vi "总磷总氮测量数据储存.vi"   [LabVIEW 2016, in "斯坦道氨氮V2.lvlib"]
uses:
  <vilib>/ptbypt/NI_PtbyPt.lvlib
types:
  T1 = cluster{"跨度值":dbl, "零点标准液浓度":dbl, "跨度标准液浓度":dbl, "标准液标准浓度":dbl}
  T2 = cluster{"系统时间":timestamp, "工作状态":u16, "测量模式":enum16{"待机", "连续模式", "周期模式", "定点模式", "受控模式", "手动模式"}, "告警代码":u16, "故障代码":u16, "日志代码":u16, "软件版本":u16, "F0":sgl, "F1":sgl, "F2":sgl, "F3":sgl, "T":sgl, "H":sgl, "id":u16, "flowid":u16, "量程":u16, "总磷控温温度1":sgl, "营养盐控温温度2":sgl, "ADC":sgl}
  T3 = cluster{"运行模式":enum16{"维护模式", "常规模式", "应急模式", "质控模式"}, "质控频次":enum16{"关闭", "每天", "星期一", "星期二", "星期三", "星期四", "星期五", "星期六", "星期日"}, "空白核查时间":u16, "跨度核查时间":u16, "测量间隔":dbl}
  T4 = cluster{"总磷跨度值":dbl, "总磷零点标准液浓度":dbl, "总磷跨度标准液浓度":dbl, "总磷标准液标准浓度":dbl, "总氮跨度值":dbl, "总氮零点标准液浓度":dbl, "总氮跨度标准液浓度":dbl, "总氮标准液标准浓度":dbl, "氨氮跨度值":dbl, "氨氮零点标准液浓度":dbl, "氨氮跨度标准液浓度":dbl, "氨氮标准液标准浓度":dbl}
  T5 = cluster{"因子编码":u32, "单位":u16, "标样参考值":sgl, "水样数据时间":timestamp, "水样实测值":sgl, "水样数据标识":string, "标样数据时间":timestamp, "标样实测值":sgl, "标样数据标识":string, "空白数据时间":timestamp, "空白实测值":sgl, "空白数据标识":string, "零点核查数据时间":timestamp, "零点核查实测值":sgl, "零点核查数据标识":string, "跨度核查数据时间":timestamp, "跨度核查实测值":sgl, "跨度核查数据标识":string, "加标回收数据时间":timestamp, "加标回收实测值":sgl, "加标回收数据标识":string, "平行样数据时间":timestamp, "平行样实测值":sgl, "平行样数据标识":string, "F0":sgl, "F1":sgl, "F2":sgl, "F3":sgl, "F4":sgl, "F5":sgl, "F6":sgl, "F7":sgl, "温度":sgl, "湿度":sgl, "X值":sgl, "fidrange":u16}[]
  T6 = cluster{"因子编码":u32, "单位":u16, "标样参考值":sgl, "水样数据时间":timestamp, "水样实测值":sgl, "水样数据标识":string, "标样数据时间":timestamp, "标样实测值":sgl, "标样数据标识":string, "空白数据时间":timestamp, "空白实测值":sgl, "空白数据标识":string, "零点核查数据时间":timestamp, "零点核查实测值":sgl, "零点核查数据标识":string, "跨度核查数据时间":timestamp, "跨度核查实测值":sgl, "跨度核查数据标识":string, "加标回收数据时间":timestamp, "加标回收实测值":sgl, "加标回收数据标识":string, "平行样数据时间":timestamp, "平行样实测值":sgl, "平行样数据标识":string, "F0":sgl, "F1":sgl, "F2":sgl, "F3":sgl, "F4":sgl, "F5":sgl, "F6":sgl, "F7":sgl, "温度":sgl, "湿度":sgl, "X值":sgl, "fidrange":u16}
  T7 = cluster{"时间标识":timestamp, "测量模式":enum16{"维护数据", "水样测试", "标样核查", "零点核查", "跨度核查", "空白测试", "平行样测试", "加标回收", "空白校准", "标样校准", "初始化（清洗）", "快捷测试"}, "数据标记表":string, "监测值":sgl, "单位":u16, "数据标识":string, "因子编码":u32, "标样参考值":sgl, "F0":sgl, "F1":sgl, "F2":sgl, "F3":sgl, "F4":sgl, "F5":sgl, "F6":sgl, "F7":sgl, "X":sgl, "温度":sgl, "湿度":sgl, "量程标识":string, "SN":string, "跨度值":sgl, "X1":sgl}
  T8 = typedef "斯坦道氨氮V2.lvlib/关键参数.ctl" = cluster{"测量量程":sgl, "测量检出限":sgl, "测量精度":sgl, "测量间隔":sgl, "消解温度":sgl, "消解时长":sgl, "三项式系数":sgl, "二次多项式系数":sgl, "曲线斜率":sgl, "曲线截距":sgl, "线性相关系数":sgl, "空白校准时间":timestamp, "标样校准时间":timestamp, "测量信号值":sgl, "稀释倍数":sgl, "空白标定系数":sgl, "量程系数":sgl}
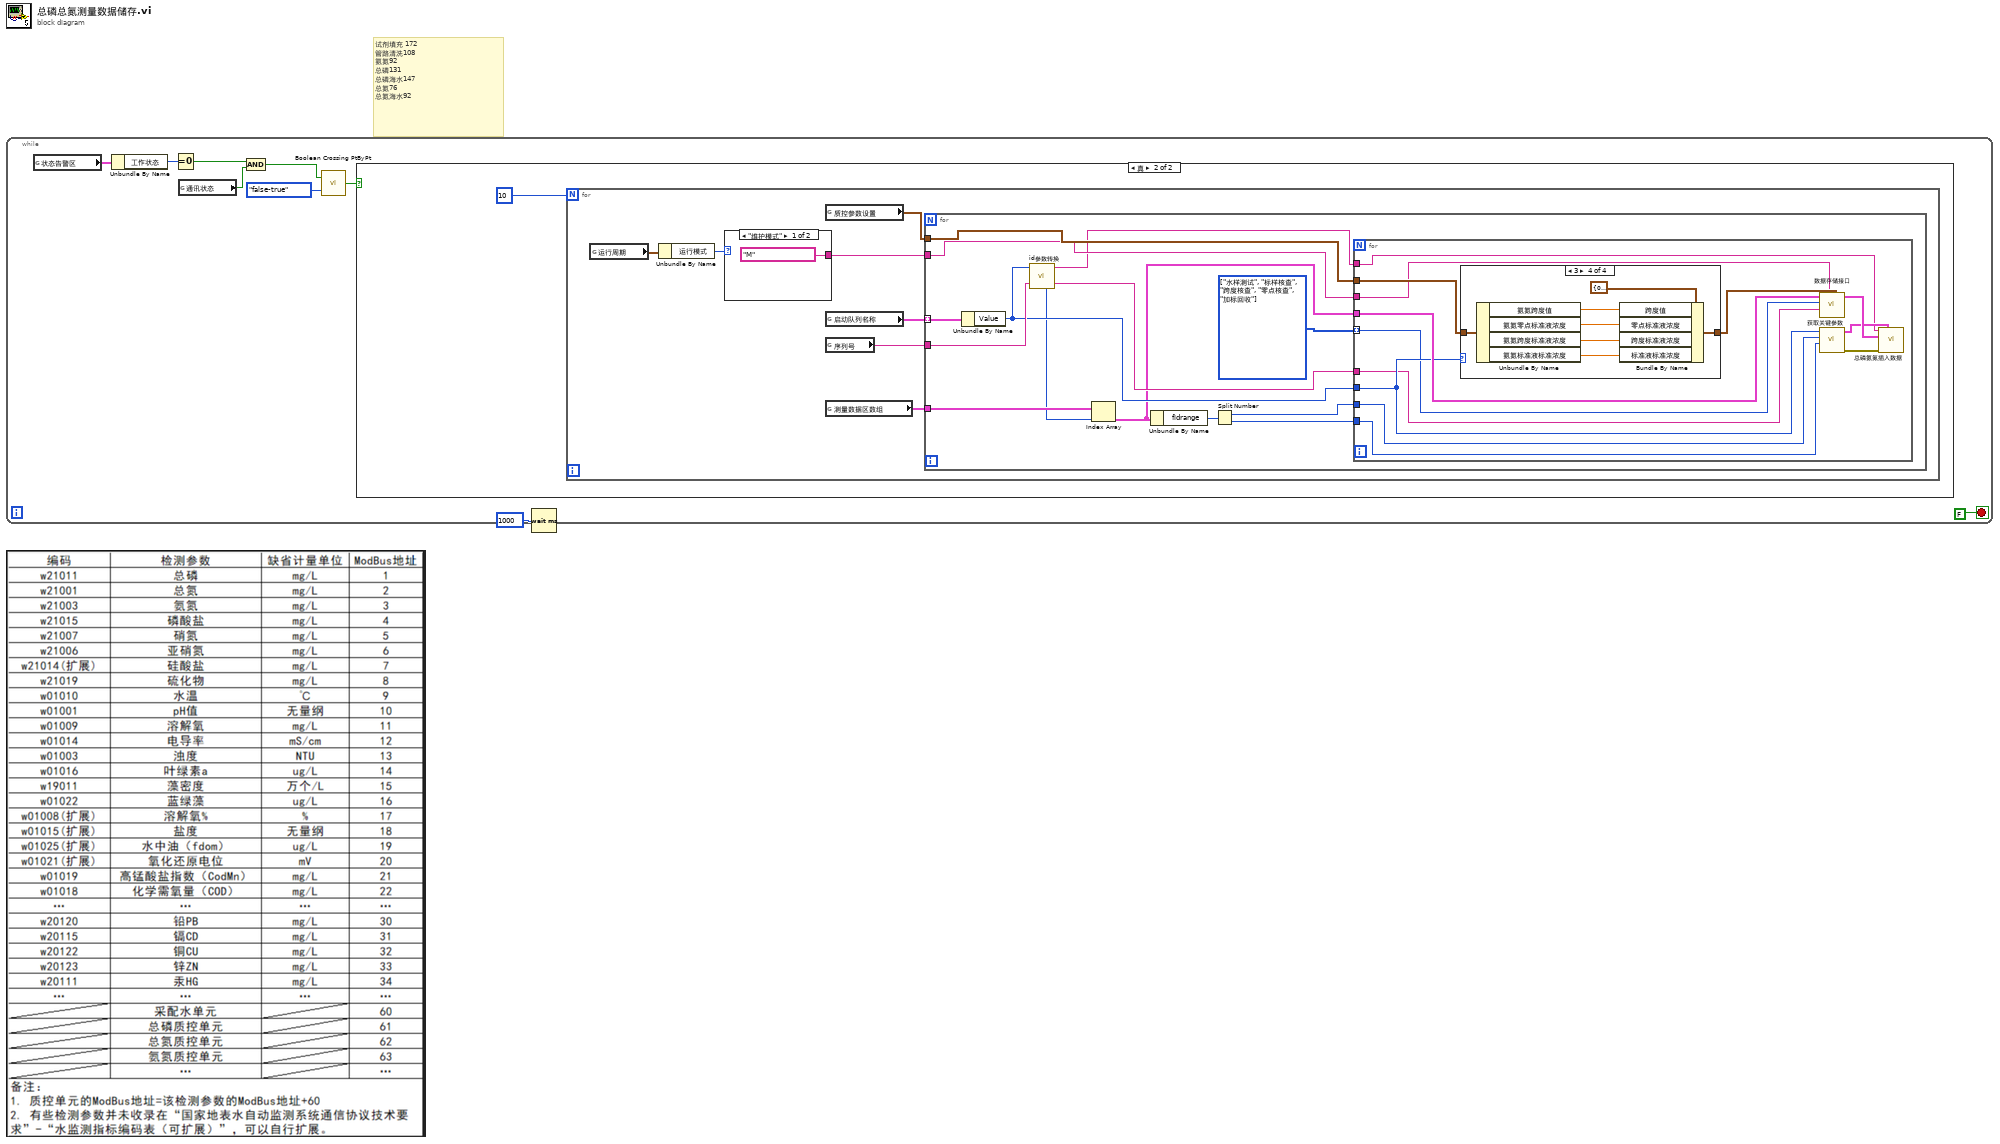
[diagram p0: block diagram]
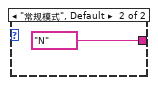
[diagram p3: hidden frame]
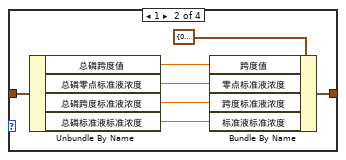
[diagram p5: hidden frame]
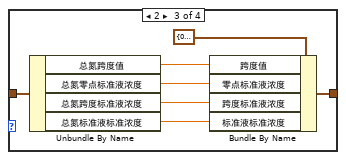
[diagram p6: hidden frame]
diagram:
  # "试剂填充 172 \n管路清洗108\n氨氮92\n总磷131\n总磷海水147\n总氮76\n总氮海水92"
  n1 = while {
    stop <- FALSE stop-if-true
    n2 = global read "VAR总磷总氮全局变量.vi" "状态告警区"() -> (w8:T2)
    n3 = Unbundle By Name(w8) -> ("工作状态"=w6:u16)
    n4 = Equal To 0?(x=w6) -> (x = 0?=w5:bool)
    n5 = global read "VAR总磷总氮全局变量.vi" "通讯状态"() -> (w4:bool)
    n6 = And(x=w5, y=w4) -> (x .and. y?=w3:bool)
    n7 = call <vilib>:"Boolean Crossing PtByPt.vi"("direction"=enum16{"either", "false-true", "true-false"}."false-true", "input"=w3) -> ("crossing"=w1:bool)  [unwired: 1 in]
    n8 = case shown="真" w1 {
      frame False {
      }
      frame True {
        n9 = for {
          N: 10 -> [_]
          n10 = global read "总磷总氮断电保存全局变量.vi" "运行周期"() -> (w12:T3)
          n11 = Unbundle By Name(w12) -> ("运行模式"=w13:enum16{"维护模式", "常规模式", "应急模式", "质控模式"})
          n12 = case shown="\"维护模式\"" w13 {
            tunnel: ["M" ("数据标记表") "N" ("数据标记表")] -> w11
            frame "维护模式" {
            }
            frame "常规模式", Default {
            }
          }
          n13 = global read "总磷总氮断电保存全局变量.vi" "质控参数设置"() -> (w17:T4)
          n14 = global read "总磷总氮断电保存全局变量.vi" "启动队列名称"() -> (w15:cluster{"String":string, "Value":u16}[])
          n15 = global read "VAR总磷总氮全局变量.vi" "序列号"() -> (w16:string)
          n16 = global read "VAR总磷总氮全局变量.vi" "测量数据区数组"() -> (w14:T5)
          n17 = for {
            tunnel: w17 -> [w32]
            tunnel: w11 -> [w30]
            tunnel: w16 -> [w29]
            tunnel: w15 -> [w28] mode=indexing
            tunnel: w14 -> [w25]
            w31 = enum16{"水样测试", "标样核查", "跨度核查", "零点核查", "加标回收"}[] [enum."水样测试", enum."标样核查", enum."跨度核查", enum."零点核查", enum."加标回收"] items=["水样测试", "标样核查", "跨度核查", "零点核查", "加标回收"]
            n18 = Unbundle By Name(w28) -> ("Value"=w27:u16)
            n19 = call "id参数转换.vi"("id"=w27) -> ("table输出"=w26:string, "数组资源索引"=w24:i32)  [unwired: 9 in]
            n20 = Index Array(array=w25, index=w24) -> (element=w22:T6)
            n21 = Unbundle By Name(w22) -> ("fidrange"=w23:u16)
            n22 = Split Number(x=w23) -> (hi(x)=w21:u8, lo(x)=w20:u8)
            n23 = for {
              tunnel: w32 -> [w44]
              tunnel: w22 -> [w40]
              tunnel: w21 -> [w39]
              tunnel: w20 -> [w38]
              tunnel: w27 -> [w37]
              tunnel: w26 -> [w36]
              tunnel: w31 -> [w35] mode=indexing
              tunnel: w30 -> [w34]
              tunnel: w29 -> [w33]
              n24 = case shown="3" w37 {
                tunnel: w44 -> [_ w52 w59 w66]
                tunnel: [_ w50 w57 w64] -> w43
                frame 0, Default {
                }
                frame 1 {
                  n25 = Unbundle By Name(w52) -> ("总磷跨度值"=w49:dbl, "总磷零点标准液浓度"=w48:dbl, "总磷跨度标准液浓度"=w47:dbl, "总磷标准液标准浓度"=w46:dbl)
                  n26 = Bundle By Name(cluster=T1 {"跨度值"=0.0, "零点标准液浓度"=0.0, "跨度标准液浓度"=0.0, "标准液标准浓度"=0.0} ("质控参数设置"), "跨度值"=w49, "零点标准液浓度"=w48, "跨度标准液浓度"=w47, "标准液标准浓度"=w46) -> (w50:T1)
                }
                frame 2 {
                  n27 = Unbundle By Name(w59) -> ("总氮跨度值"=w56:dbl, "总氮零点标准液浓度"=w55:dbl, "总氮跨度标准液浓度"=w54:dbl, "总氮标准液标准浓度"=w53:dbl)
                  n28 = Bundle By Name(cluster=T1 {"跨度值"=0.0, "零点标准液浓度"=0.0, "跨度标准液浓度"=0.0, "标准液标准浓度"=0.0} ("质控参数设置"), "跨度值"=w56, "零点标准液浓度"=w55, "跨度标准液浓度"=w54, "标准液标准浓度"=w53) -> (w57:T1)
                }
                frame 3 {
                  n29 = Unbundle By Name(w66) -> ("氨氮跨度值"=w63:dbl, "氨氮零点标准液浓度"=w62:dbl, "氨氮跨度标准液浓度"=w61:dbl, "氨氮标准液标准浓度"=w60:dbl)
                  n30 = Bundle By Name(cluster=T1 {"跨度值"=0.0, "零点标准液浓度"=0.0, "跨度标准液浓度"=0.0, "标准液标准浓度"=0.0} ("质控参数设置"), "跨度值"=w63, "零点标准液浓度"=w62, "跨度标准液浓度"=w61, "标准液标准浓度"=w60) -> (w64:T1)
                }
              }
              n31 = call "数据存储接口.vi"("质控参数设置"=w43, "数据标记表"=w34, "SN"=w33, "数据存储模式"=w35, "测量数据区"=w40) -> ("data输出"=w45:T7)  [unwired: 6 in]
              n32 = call "获取关键参数.vi"("量程"=w38, "flowid"=w39, "id"=w37) -> ("error out"=w42:errorcluster, "关键参数"=w41:T8)  [unwired: 7 in]
              n33 = call "总磷氨氮插入数据.vi"("table"=w36, "关键参数"=w41, "data"=w45, "error in (no error)"=w42) -> ()  [unwired: 11 in, 1 out]
            }
          }
        }
      }
    }
    n34 = Wait (ms)(milliseconds to wait=u32 1000 ("等待时间（毫秒）")) -> ()  [unwired: 1 out]
  }
